vi "PH_Revolver-GUI_6P.set i attribute.vi"(0 "i ref in":refnum<vi>, 2 "i attribute":T1={"GUI Refs"={"0°"=refnum, "60°"=refnum, "120°"=refnum, "180°"=refnum, "240°"=refnum, "300°"=refnum, "Action"=refnum}, "Revolver Position"=0, "Service ID Position"=-1, "Captions"=[]} {"Revolver Position" items=["unknown", "Position 0", "Position 60", "Position 120", "Position 180", "Position 240", "Position 300", "moving"]}, 5 "error in (no error)":errorcluster) -> (14 "i ref out":refnum<vi>, 19 "error out":errorcluster)   [LabVIEW 2014, in "PH_Revolver-GUI_6P.lvlib"]
doc: "Sets the i attribute data of an object.\n\nLicense Agreement for this software:\n\nCopyright (C)\nGesellschaft für Schwerionenforschung, GSI\nPlanckstr. 1\n64291 Darmstadt\nGermany\n\nContact: D.Beck@gsi.de \n\nThis program is free software; you can redistribute it and/or modify it under the terms of the GNU General Public License as published by the Free Software Foundation; either version 2 of the license, or (at your option) any later version.\n\nThis program is distributed in the hope that it will be useful, but WITHOUT ANY WARRANTY; without even the implied warranty of MERCHANTABILITY or FITNESS FOR A PARTICULAR PURPOSE. See the GNU General License for more details (http://www.gnu.org).\n\nGesellschaft für Schwerionenforschung, GSI\nPlanckstr. 1, 64291 Darmstadt, Germany\nFor all questions and ideas contact: M.Richter@gsi.de, H.Brand@gsi.de or D.Beck@gsi.de.\nLast update: 17-JUN-2004"
uses:
  PH_Revolver-GUI_6P.lvlib
  PH_Revolver-GUI_6P.i attribute.ctl
  PH_Revolver-GUI_6P.Position.ctl
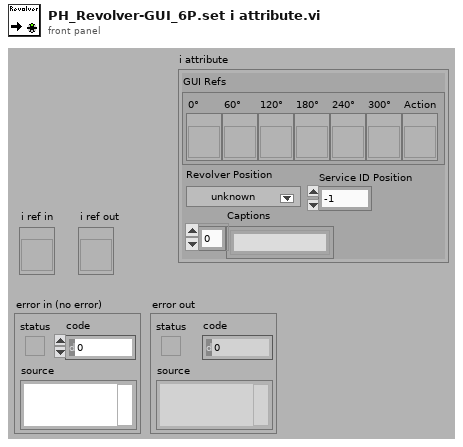
[diagram p1: front panel]
types:
  T1 = typedef "PH_Revolver-GUI_6P.lvlib/PH_Revolver-GUI_6P.i attribute.ctl" = cluster{"GUI Refs":cluster{"0°":refnum<vi>, "60°":refnum<vi>, "120°":refnum<vi>, "180°":refnum<vi>, "240°":refnum<vi>, "300°":refnum<vi>, "Action":refnum<vi>}, "Revolver Position":T2, "Service ID Position":i32, "Captions":string[]}
  T2 = typedef "PH_Revolver-GUI_6P.lvlib/PH_Revolver-GUI_6P.Position.ctl" = u16
  T3 = enum16{"SetAttribute", "GetAttribute", "CreateAttribute", "DestroyAttribute", "DestroyAllAtributes"}
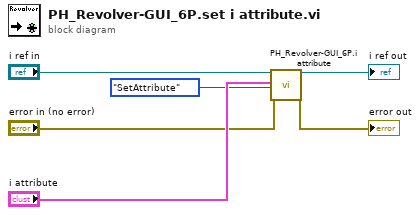
[diagram p0: block diagram]
diagram:
  n1 = call "PH_Revolver-GUI_6P.i attribute.vi"("VI Refnum"="i ref in", "CLASS.i attribute"="i attribute", "Action"=T3."SetAttribute", "error in (no error)"="error in (no error)") -> ("VI Refnum out"=→"i ref out":refnum<vi>, "error out"=→"error out":errorcluster)  [unwired: 13 in, 1 out]
